vi "Get_Process is finish.vi"(8 "error in (no error)":errorcluster caption="entrée d'erreur (pas d'erreur)", 11 "Process (Default) en entrée":refnum<class "Process (Default).lvclass">) -> (0 "error out":errorcluster caption="sortie d'erreur", 2 "Process is finish":bool, 3 "Process (Default) en sortie":refnum<class "Process (Default).lvclass">)   [LabVIEW 2020, in "Library Instrument & Equipement.lvlib" / "Process (Default).lvclass"]
uses:
  Process (Default).lvclass
  Process (Default).lvclass/Process (Default).ctl
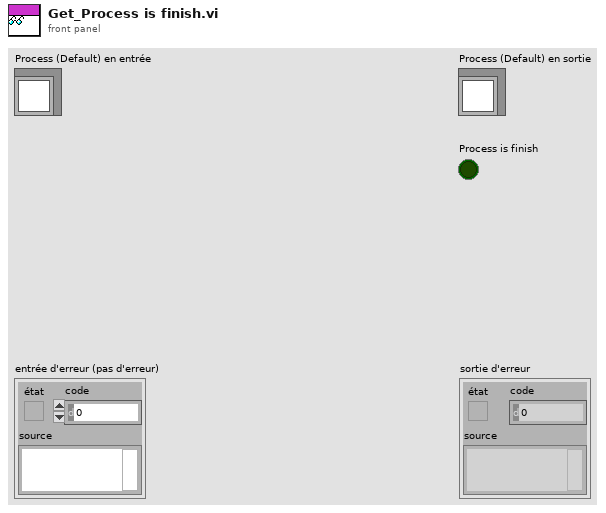
[diagram p1: front panel]
types:
  T1 = cluster{"Standard Output":string, "Process_is_Finish":bool}
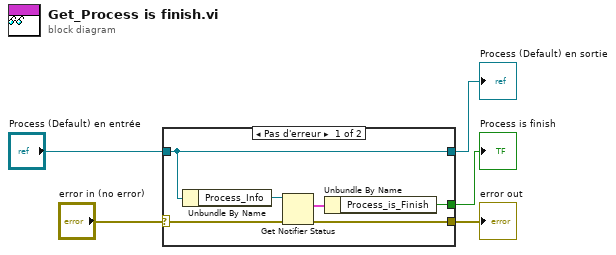
[diagram p0: block diagram]
diagram:
  n1 = case shown="Pas d'erreur" "error in (no error)" {
    selector: "error in (no error)" -> [w7 w12]
    tunnel: [w6 w12] -> w2
    tunnel: [w11 w13] -> w1
    tunnel: "Process (Default) en entrée" -> [w11 w13]
    tunnel: [w8 _] -> w3
    frame No Error {
      n2 = Unbundle By Name(w11) -> ("Process_Info"=w10:refnum<notifier>)
      n3 = Get Notifier Status(notifier=w10, error in (no error)=w7) -> (current notification=w9:T1, error out=w6:errorcluster)  [unwired: 3 out]
      n4 = Unbundle By Name(w9) -> ("Process_is_Finish"=w8:bool)
    }
    frame Error {
    }
  }
  "error out" <- w2
  "Process (Default) en sortie" <- w1
  "Process is finish" <- w3
